vi "Graphs.vi"() -> (9 "Waveform Chart":dbl(graph), 10 "XY Graph":cluster{dbl, dbl}[](graph), 11 "Waveform Graph":dbl[](graph))   [LabVIEW 2012]
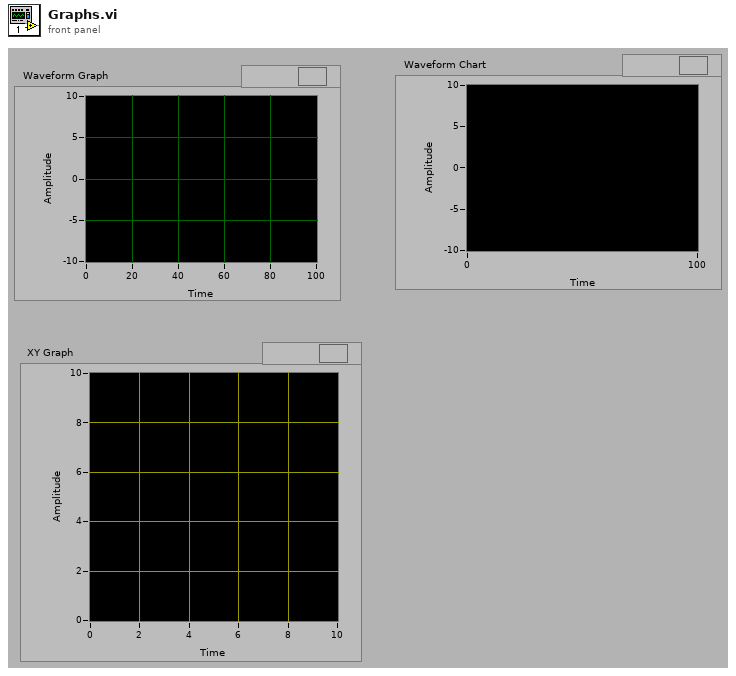
[diagram p1: front panel]
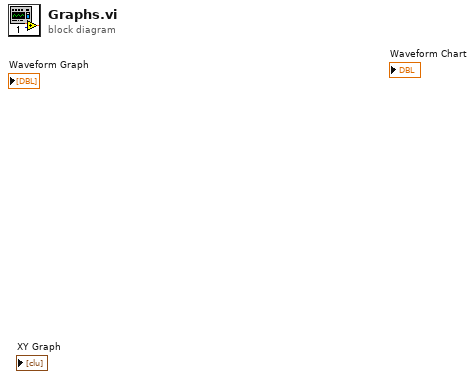
[diagram p0: block diagram]
diagram:
